vi "VIP Prebuild.vi"() -> ()   [LabVIEW 2020]
uses:
  dev/Tags.ctl
panel:
  out "Next Version":string
  # "Run this VI before building a new VIPM package. Ensure the VIPB has been saved before running this VI, the VIPB can be open while this is run.\n\nAfter running this VI the Next Version indicator above should match the Version Number of Next Build fields in VIPB for the package."
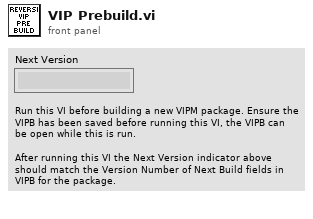
[diagram p1: front panel]
types:
  T1 = typedef "Tags.ctl" = enum16{"sol.reversi.version"}
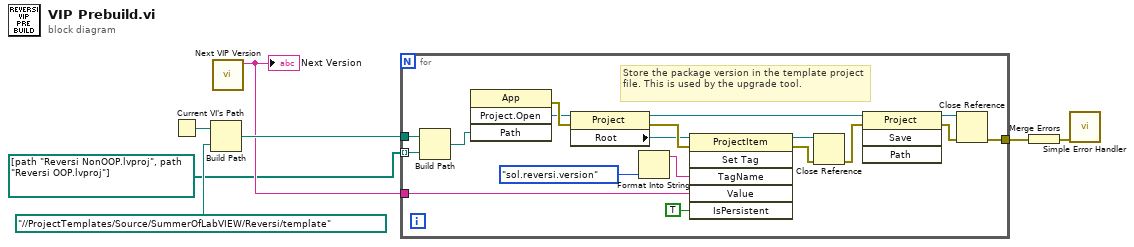
[diagram p0: block diagram]
diagram:
  n1 = Current VI's Path() -> (path=w7:path)
  n2 = Build Path(base path=w7, name or relative path=path "../../ProjectTemplates/Source/SummerOfLabVIEW/Reversi/template") -> (appended path=w4:path)
  n3 = call "Next VIP Version.vi"() -> ("Next Version"=w3:string)  [unwired: 10 in, 1 out]
  "Next Version" <- w3
  n4 = for {
    tunnel: [w14] -> w5
    tunnel: w4 -> [w11]
    tunnel: w3 -> [w10]
    tunnel: path[] [path "Reversi NonOOP.lvproj", path "Reversi OOP.lvproj"] -> [w9] mode=indexing
    # "Store the package version in the template project file. This is used by the upgrade tool."
    n5 = Build Path(base path=w11, name or relative path=w9) -> (appended path=w13:path)
    n6 = invoke class="App" method="Project.Open"("Path"=w13) -> (error out=w25:errorcluster, "Project:Open"=w22:refnum<vi>)  [unwired: 3 in, 2 out]
    n7 = property class="Project"(reference=w22, error in=w25) -> (reference out=w23:refnum<vi>, error out=w24:errorcluster, "Root"=w21:refnum<vi>)
    n8 = Format Into String(Tags."sol.reversi.version" ("Tags")) -> (resulting string=w12:string)  [unwired: 3 in, 1 out]
    n9 = invoke class="ProjectItem" method="Set Tag"(reference=w21, error in=w24, "TagName"=w12, "Value"=w10, "IsPersistent"=TRUE ("Is Persistent (T)")) -> (reference out=w19:refnum<vi>, error out=w18:errorcluster)  [unwired: 1 in, 4 out]
    n10 = Close Reference(reference=w19, error in (no error)=w18) -> (error out=w17:errorcluster)
    n11 = invoke class="Project" method="Save"(reference=w23, error in=w17) -> (reference out=w16:refnum<vi>, error out=w15:errorcluster)  [unwired: 2 in, 2 out]
    n12 = Close Reference(reference=w16, error in (no error)=w15) -> (error out=w14:errorcluster)
  }
  n13 = Merge Errors(w5) -> (w2:errorcluster)
  n14 = call <vilib>:"Simple Error Handler.vi"("error in (no error)"=w2) -> ()  [unwired: 4 in, 5 out]
